vi "Bundle Tabs.vi"(10 "tab ref 2":refnum<vi>, 11 "tab ref 1":refnum<vi>) -> (3 "tab references":T1)   [LabVIEW 2020]
uses:
  Tab Reference.ctl
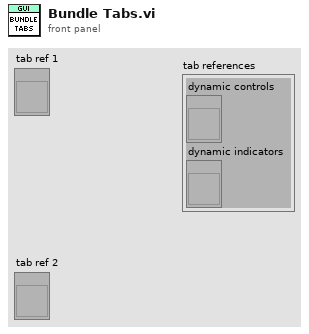
[diagram p1: front panel]
types:
  T1 = typedef "Tab Reference.ctl" = cluster{"dynamic controls":refnum<vi>, "dynamic indicators":refnum<vi>}
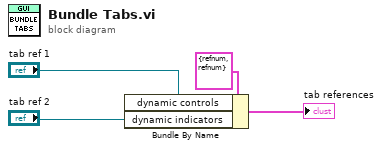
[diagram p0: block diagram]
diagram:
  n1 = Bundle By Name(cluster=T1 {"dynamic controls"=refnum, "dynamic indicators"=refnum}, "dynamic controls"="tab ref 1", "dynamic indicators"="tab ref 2") -> (→"tab references":T1)
